vi "Alazar_ChannelConfig.vi"(3 "Channel":u32, 4 "V scale":T1 {"Coupling" items=["DC 1 MOhm", "AC 1 MOhm", "DC 50 Ohm", "AC 50 OHM"]; "Offset" format="%.2f"}, 5 "DeviceIn":u32) -> (0 "Return":u32, 1 "Handle_Out":u32, 2 "DeviceOut":u32)   [LabVIEW 2022 SP3]
uses:
  C:/AlazarTech/ATS-VI/6.2.0/ATS_ctl/Coupling.ctl
  C:/AlazarTech/ATS-VI/6.2.0/ATS_ctl/Impedance.ctl
  C:/AlazarTech/ATS-VI/6.2.0/ATS_ctl/Device_Ctrl.ctl
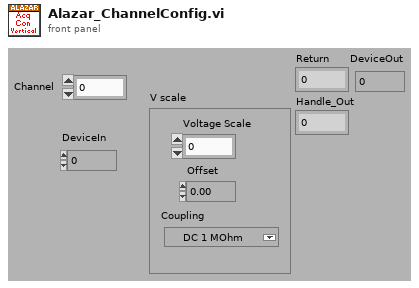
[diagram p1: front panel]
types:
  T1 = cluster{"Voltage Scale":dbl, "Offset":dbl, "Coupling":u16}
  T2 = typedef "Device_Ctrl.ctl" = enum16{"Status", "About", "Arm", "ForceTrig", "Abort", "Initialize", "Init (NoPreset)", "Info", "Close", "Calibrate", "SetManually", "LED_ON", "LED_OFF"}
  T3 = typedef "Coupling.ctl" = enum16{"AC", "DC"}
  T4 = typedef "Impedance.ctl" = enum16{"1M ohms", "50 ohms"}
  T5 = typedef "Device_Info.ctl" = cluster{"Handle":u32, "Board":string, "CPLD":string, "MemorySize":u32, "SampleSize":u8, "ID":i32, "High_Memory":bool, "Chan/Board":u8}
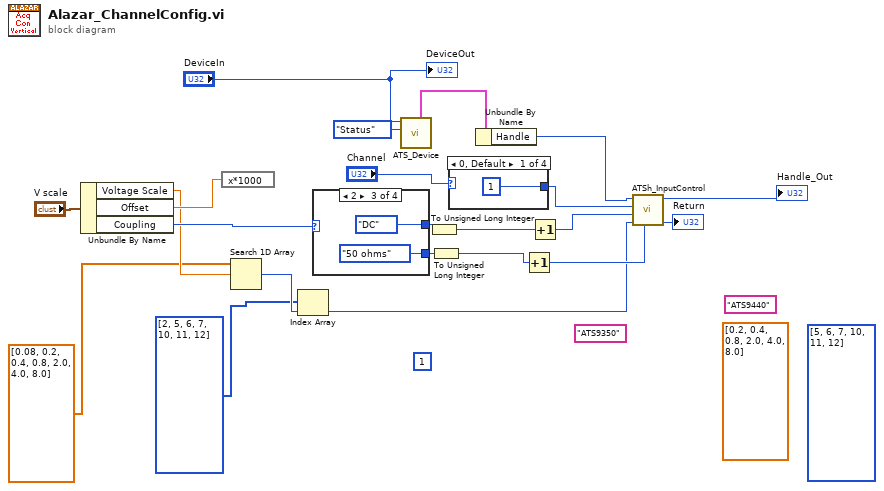
[diagram p0: block diagram]
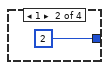
[diagram p2: hidden frame]
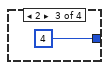
[diagram p3: hidden frame]
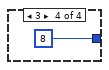
[diagram p4: hidden frame]
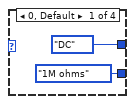
[diagram p5: hidden frame]
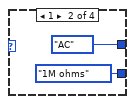
[diagram p6: hidden frame]
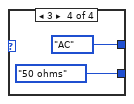
[diagram p7: hidden frame]
diagram:
  (unwired) u32 1 ("Channel")
  (unwired) "ATS9440"
  (unwired) "ATS9350"
  (unwired) dbl[] [0.2, 0.4, 0.8, 2.0, 4.0, 8.0]
  (unwired) u32[] [5, 6, 7, 10, 11, 12]
  n1 = Unbundle By Name("V scale") -> ("Voltage Scale"=w16:dbl, "Offset"=w20:dbl, "Coupling"=w21:u16)
  n2 = expression code="x*1000"(w20) -> ()  [unwired: 1 out]
  n3 = Search 1D Array(1D array=dbl[] [0.08, 0.2, 0.4, 0.8, 2.0, 4.0, 8.0], element=w16) -> (index of element=w15:i32)  [unwired: 1 in]
  n4 = Index Array(array=u32[] [2, 5, 6, 7, 10, 11, 12], index=w15) -> (element=w9:u32)
  n5 = case shown="2" w21 {
    tunnel: [Coupling."DC" ("Coupling") Coupling."AC" ("Coupling") Coupling."DC" ("Coupling") Coupling."AC" ("Coupling")] -> w13
    tunnel: [Impedance."1M ohms" ("Impedance") Impedance."1M ohms" ("Impedance") Impedance."50 ohms" ("Impedance") Impedance."50 ohms" ("Impedance")] -> w11
    frame 0, Default {
    }
    frame 1 {
    }
    frame 2 {
    }
    frame 3 {
    }
  }
  n6 = call "ATS_Device.vi"("DevCtrl"=Device_Ctrl."Status", "DeviceIn"="DeviceIn") -> ("DevInfo"=w17:T5)  [unwired: 3 in, 6 out]
  n7 = To Unsigned Long Integer(number=w13) -> (unsigned 32bit integer=w7:u32)
  n8 = To Unsigned Long Integer(number=w11) -> (unsigned 32bit integer=w6:u32)
  n9 = case shown="0, Default" "Channel" {
    tunnel: [u32 1 ("Channel") u32 2 ("Channel") u32 4 ("Channel") u32 8 ("Channel")] -> w3
    frame 0, Default {
    }
    frame 1 {
    }
    frame 2 {
    }
    frame 3 {
    }
  }
  n10 = Unbundle By Name(w17) -> ("Handle"=w14:u32)
  n11 = Increment(x=w6) -> (x+1=w10:u32)
  n12 = Increment(x=w7) -> (x+1=w12:u32)
  n13 = call "ATSh_InputControl.vi"("Impedance"=w10, "InputRange"=w9, "Coupling"=w12, "Channel"=w3, "HandleIn"=w14) -> ("Return"=→"Return":u32, "Handle_Out"=→"Handle_Out":u32)  [unwired: 4 in, 1 out]
  "DeviceOut" <- "DeviceIn"
